vi "Drive_MP.vi"(8 "Backwards?":bool, 9 "Right Motor Name":string, 10 "Left Motor Name":string, 11 "Path Name":string) -> (0 "Time to Complete":dbl, 2 "Right Side Velocity Target":dbl, 3 "Left Side Velocity Target":dbl)   [LabVIEW 2020]
uses:
  <vilib>/Rock Robotics/WPI/ThirdParty/REV Robotics/REVLib/Typedef/Spark MAX Control Type.ctl
  <vilib>/Utility/file.llb/Read Delimited Spreadsheet (DBL).vi
panel:
  out "Measured Velocity":dbl
  out "Loop Iteration":dbl
  out "Velocity Target":dbl
  out "all rows":dbl[][](array[numeric])
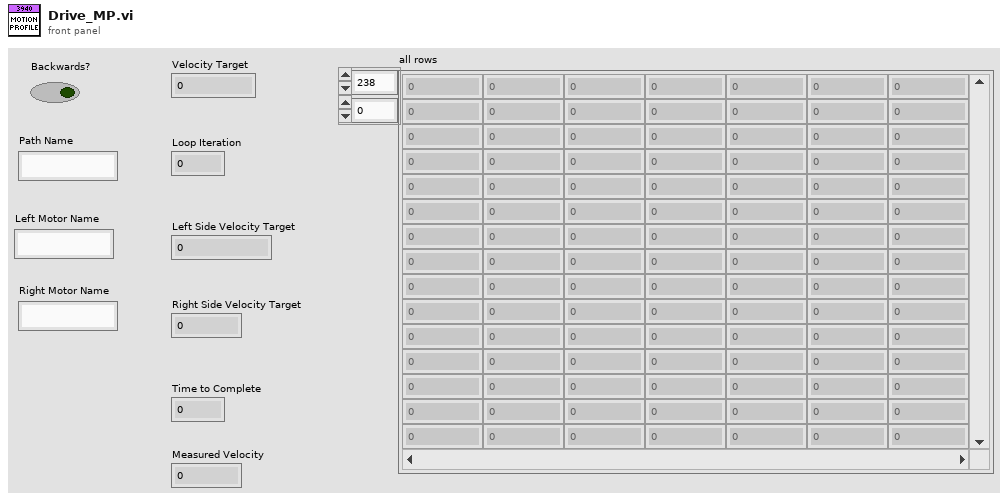
[diagram p1: front panel]
types:
  T1 = typedef "Spark MAX Control Type.ctl" = enum16{"Percent VBus", "Voltage", "Velocity", "Position", "Smart Motion", "Current", "Smart Velocity"}
  T2 = cluster{"P Gain":dbl, "I Gain":dbl, "D Gain":dbl, "F Gain":dbl, "I Zone":dbl, "Min Output":dbl, "Max Output":dbl}
  T3 = typedef "WPI_MotorControlDeviceRef.ctl" = cluster{"DeviceStatus":errorcluster, "Type":T4, "PWM":cluster{"PWM Channel":T5, "DeadBand":T6}, "CAN":cluster{"Device Number":u8, "SetOutput VI Ref":variant, "GetOutput VI Ref":variant, "Enable VI Ref":variant, "Disable VI Ref":variant, "Data":variant}, "Invert":bool, "DIO PWM":cluster{"PWM \"Enable\" Channel":T5, "DIOChannel":T7, "PWM Rate":dbl}}
  T4 = typedef "WPI_MotorControlType.ctl" = enum16{"PWM", "CAN", "DIO PWM"}
  T5 = typedef "FPGA_DIOPWMChannel.ctl" = enum8{"PWM 0", "PWM 1", "PWM 2", "PWM 3", "PWM 4", "PWM 5", "PWM 6", "PWM 7", "PWM 8", "PWM 9", "PWM MXP 0", "PWM MXP 1", "PWM MXP 2", "PWM MXP 3", "PWM MXP 4", "PWM MXP 5", "PWM MXP 6", "PWM MXP 7", "PWM MXP 8", "PWM MXP 9", "Invalid"}
  T6 = typedef "WPI_PWMDeadband.ctl" = cluster{"Name":string, "maxPositivePwm":i32, "minPositivePwm":i32, "centerPwm":i32, "maxNegativePwm":i32, "minNegativePwm":i32, "angularRange":u16}
  T7 = typedef "FPGA_DIOChannel.ctl" = enum8{"DIO 0", "DIO 1", "DIO 2", "DIO 3", "DIO 4", "DIO 5", "DIO 6", "DIO 7", "DIO 8", "DIO 9", "DIO MXP 0", "DIO MXP 1", "DIO MXP 2", "DIO MXP 3", "DIO MXP 4", "DIO MXP 5", "DIO MXP 6", "DIO MXP 7", "DIO MXP 8", "DIO MXP 9", "DIO MXP 10", "DIO MXP 11", "DIO MXP 12", "DIO MXP 13", "DIO MXP 14", "DIO MXP 15", "SPI Port CS1", "SPI Port CS2", "SPI Port CS3", "SPI Port MISO", "SPI Port MOSI", "Invalid"}
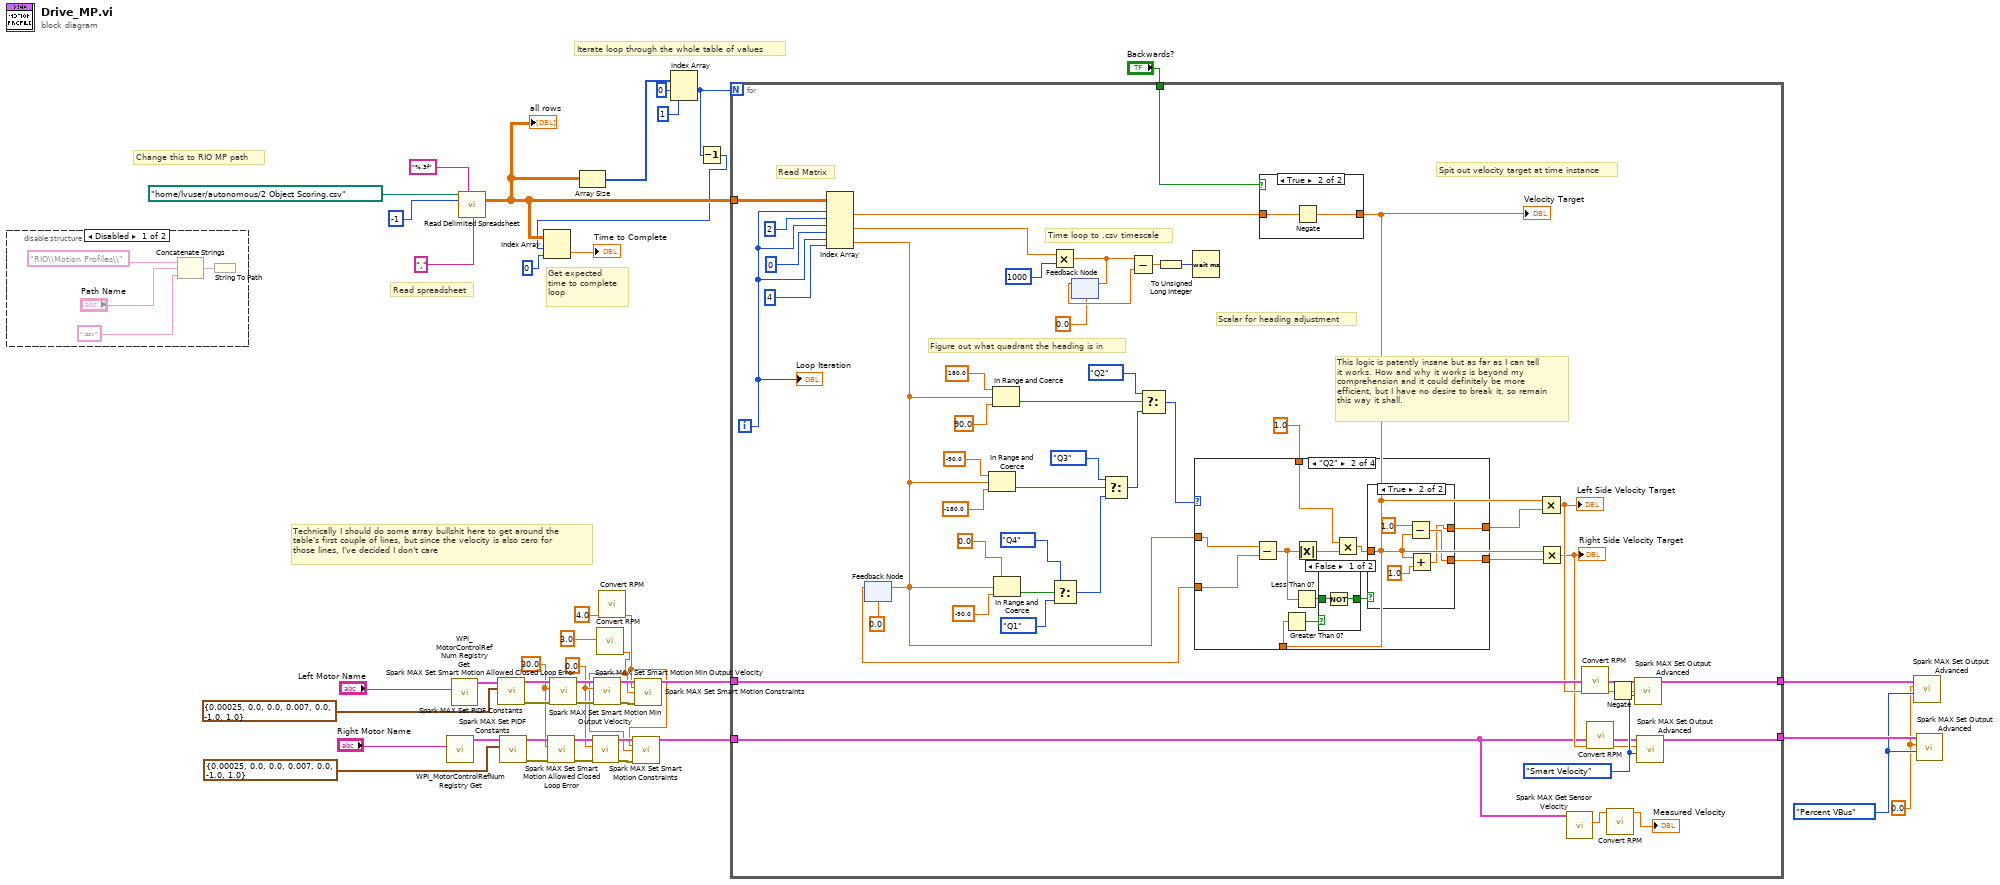
[diagram p0: block diagram]
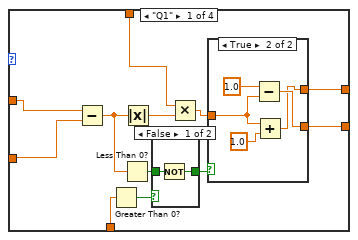
[diagram p4: hidden frame]
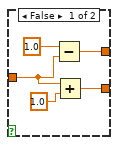
[diagram p6: hidden frame]
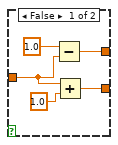
[diagram p8: hidden frame]
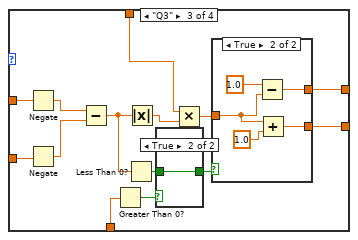
[diagram p9: hidden frame]
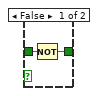
[diagram p10: hidden frame]
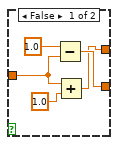
[diagram p11: hidden frame]
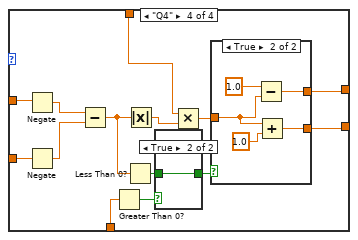
[diagram p12: hidden frame]
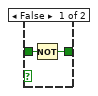
[diagram p13: hidden frame]
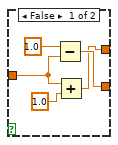
[diagram p14: hidden frame]
diagram:
  w3 = 0.0 ("Minimum Velocity Output")
  w4 = 30.0 ("Allowed Closed Loop Error")
  w21 = 0.0 ("Setpoint")
  w22 = Spark_MAX_Control_Type."Percent VBus" ("Control Mode")
  # "Get expected\ntime to complete\nloop"
  # "Change this to RIO MP path"
  # "Read spreadsheet"
  # "Iterate loop through the whole table of values"
  # "Technically I should do some array bullshit here to get around the\ntable's first couple of lines, but since the velocity is also zero for\nthose lines, I've decided I don't care"
  n1 = disable-structure shown="Disabled" {
    frame Disabled {
      n2 = Concatenate Strings("RIO\\Motion Profiles\\", "Path Name", ".csv") -> (w47:string)
      n3 = String To Path(string=w47) -> ()  [unwired: 1 out]
    }
    frame Enabled {
    }
  }
  n4 = call <vilib>:"WPI_MotorControlRefNum Registry Get.vi"("refnum name"="Right Motor Name") -> ("MotorControlDevRef"=w26:T3)  [unwired: 9 in, 1 out]
  n5 = call <vilib>:"WPI_MotorControlRefNum Registry Get.vi"("refnum name"="Left Motor Name") -> ("MotorControlDevRef"=w28:T3)  [unwired: 9 in, 1 out]
  n6 = call-poly <vilib>:"Read Delimited Spreadsheet.vi"("file path (dialog if empty)"=path "/home/lvuser/autonomous/2 Object Scoring.csv" ("file path (use dialog)"), "format (%.3f)"="%.3f", "number of rows (all:-1)"=-1, "delimiter (\\t)"="," ("delimiter (\\t)")) -> ("all rows"=w35:dbl[][])  [unwired: 6 in, 5 out]
  "all rows" <- w35
  n7 = call <vilib>:"Spark MAX Set PIDF Constants.vi"("PID Constants"=T2 {"P Gain"=0.00025, "I Gain"=0.0, "D Gain"=0.0, "F Gain"=0.007, "I Zone"=0.0, "Min Output"=-1.0, "Max Output"=1.0}, "MotorControlDeviceRef"=w28) -> ("error out"=w20:errorcluster, "MotorControlDeviceRef"=w19:T3)  [unwired: 8 in]
  n8 = call <vilib>:"Spark MAX Set PIDF Constants.vi"("PID Constants"=T2 {"P Gain"=0.00025, "I Gain"=0.0, "D Gain"=0.0, "F Gain"=0.007, "I Zone"=0.0, "Min Output"=-1.0, "Max Output"=1.0}, "MotorControlDeviceRef"=w26) -> ("error out"=w9:errorcluster, "MotorControlDeviceRef"=w10:T3)  [unwired: 8 in]
  n9 = call <vilib>:"Spark MAX Set Smart Motion Allowed Closed Loop Error.vi"("error in"=w9, "Allowed Closed Loop Error"=w4, "MotorControlDeviceRef"=w10) -> ("error out"=w12:errorcluster, "MotorControlDeviceRef"=w8:T3)  [unwired: 7 in]
  n10 = call <vilib>:"Spark MAX Set Smart Motion Allowed Closed Loop Error.vi"("error in"=w20, "Allowed Closed Loop Error"=w4, "MotorControlDeviceRef"=w19) -> ("error out"=w18:errorcluster, "MotorControlDeviceRef"=w17:T3)  [unwired: 7 in]
  n11 = Array Size(array=w35) -> (size(s)=w40:i32[])
  n12 = call <vilib>:"Spark MAX Set Smart Motion Min Output Velocity.vi"("error in"=w12, "Minimum Velocity Output"=w3, "MotorControlDeviceRef"=w8) -> ("error out"=w11:errorcluster, "MotorControlDeviceRef"=w7:T3)  [unwired: 7 in]
  n13 = call <vilib>:"Spark MAX Set Smart Motion Min Output Velocity.vi"("error in"=w18, "Minimum Velocity Output"=w3, "MotorControlDeviceRef"=w17) -> ("error out"=w15:errorcluster, "MotorControlDeviceRef"=w16:T3)  [unwired: 7 in]
  n14 = call "Convert RPM.vi"("Velocity (m/s)"=3.0) -> ("Velocity (RPM)"=w2:dbl)  [unwired: 9 in, 1 out]
  n15 = call "Convert RPM.vi"("Velocity (m/s)"=4.0) -> ("Velocity (RPM)"=w1:dbl)  [unwired: 9 in, 1 out]
  n16 = call <vilib>:"Spark MAX Set Smart Motion Constraints.vi"("MotorControlDeviceRef"=w7, "Max Velocity"=w1, "Max Acceleration"=w2, "error in"=w11) -> ("MotorControlDeviceRef"=w6:T3)  [unwired: 10 in, 1 out]
  n17 = call <vilib>:"Spark MAX Set Smart Motion Constraints.vi"("MotorControlDeviceRef"=w16, "Max Velocity"=w1, "Max Acceleration"=w2, "error in"=w15) -> ("MotorControlDeviceRef"=w5:T3)  [unwired: 10 in, 1 out]
  n18 = Index Array(array=w40, index #1=0 ("index"), index #2=1 ("index")) -> (element #1=w32:i32)  [unwired: 1 out]
  n19 = Decrement(x=w32) -> (x-1=w31:i32)
  n20 = Index Array(array=w35, index (row)=w31, index (col)=0 ("disabled index (col)")) -> (element=→"Time to Complete":dbl)
  n21 = for {
    N: w32 -> [_]
    tunnel: w35 -> [w96]
    tunnel: "Backwards?" -> [w60]
    tunnel: w5 -> [w59]
    tunnel: w6 -> [w51]
    tunnel: [w58] -> w24
    tunnel: [w57] -> w23
    i -> [w86]
    w56 = Spark_MAX_Control_Type."Smart Velocity" ("Control Mode")
    # "This logic is patently insane but as far as I can tell\nit works. How and why it works is beyond my\ncomprehension and it could definitely be more\nefficient, but I have no desire to break it, so remain\nthis way it shall."
    # "Scalar for heading adjustment"
    # "Figure out what quadrant the heading is in"
    # "Time loop to .csv timescale"
    # "Spit out velocity target at time instance"
    # "Read Matrix"
    n22 = Index Array(array=w96, index (row) #1=w86, index (col) #1=2 ("disabled index (col)"), index (row) #2=w86, index (col) #2=0 ("disabled index (col)"), index (row) #3=w86, index (col) #3=4 ("disabled index (col)")) -> (element #1=w62:dbl, element #2=w92:dbl, element #3=w67:dbl)
    n23 = feedback #1(0.0 ("Numeric")) -> (w68:dbl)
    n24 = feedback-in #1(w67) -> ()
    n25 = In Range and Coerce(upper limit=-90.0, x=w67, lower limit=-180.0) -> (In Range?=w78:bool)  [unwired: 1 out]
    n26 = In Range and Coerce(upper limit=180.0, x=w67, lower limit=90.0) -> (In Range?=w82:bool)  [unwired: 1 out]
    n27 = In Range and Coerce(upper limit=0.0, x=w67, lower limit=-90.0) -> (In Range?=w74:bool)  [unwired: 1 out]
    n28 = Multiply(x=w92, y=1000) -> (x*y=w88:dbl)
    n29 = Select(t=enum16{"Q1", "Q2", "Q3", "Q4"}."Q4", s=w74, f=enum16{"Q1", "Q2", "Q3", "Q4"}."Q1") -> (s? t:f=w71:enum16{"Q1", "Q2", "Q3", "Q4"})
    n30 = feedback #2(0.0) -> (w89:dbl)
    n31 = feedback-in #2(w88) -> ()
    n32 = Select(t=enum16{"Q1", "Q2", "Q3", "Q4"}."Q3", s=w78, f=w71) -> (s? t:f=w72:enum16{"Q1", "Q2", "Q3", "Q4"})
    n33 = Subtract(x=w88, y=w89) -> (x-y=w90:dbl)
    n34 = Select(t=enum16{"Q1", "Q2", "Q3", "Q4"}."Q2", s=w82, f=w72) -> (s? t:f=w69:enum16{"Q1", "Q2", "Q3", "Q4"})
    n35 = To Unsigned Long Integer(number=w90) -> (unsigned 32bit integer=w91:u32)
    n36 = Wait (ms)(milliseconds to wait=w91) -> ()  [unwired: 1 out]
    n37 = case shown="True" w60 {
      tunnel: w62 -> [w97 w99]
      tunnel: [w97 w98] -> w61
      frame False {
      }
      frame True {
        n38 = Negate(x=w99) -> (-x=w98:dbl)
      }
    }
    "Velocity Target" <- w61
    n39 = case shown="\"Q2\"" w69 {
      tunnel: w68 -> [w103 w125 w162 w178]
      tunnel: w67 -> [w104 w126 w163 w179]
      tunnel: [w100 w129 w158 w181] -> w65
      tunnel: [w101 w128 w157 w180] -> w64
      tunnel: 1.0 ("x") -> [w105 w130 w154 w182]
      tunnel: w61 -> [w102 w127 w153 w177]
      frame "Q1" {
        n40 = Subtract(x=w104, y=w103) -> (x-y=w111:dbl)
        n41 = Greater Than 0?(x=w102) -> (x > 0?=w108:bool)
        n42 = Less Than 0?(x=w111) -> (x < 0?=w107:bool)
        n43 = Absolute Value(x=w111) -> (abs(x)=w110:dbl)
        n44 = case shown="False" w108 {
          tunnel: w107 -> [w113 w114]
          tunnel: [w112 w114] -> w106
          frame False {
            n45 = Not(x=w113) -> (.not. x?=w112:bool)
          }
          frame True {
          }
        }
        n46 = Multiply(x=w105, y=w110) -> (x*y=w109:dbl)
        n47 = case shown="True" w106 {
          tunnel: w109 -> [w117 w121]
          tunnel: [w116 w120] -> w100
          tunnel: [w115 w122] -> w101
          frame False {
            n48 = Subtract(x=1.0, y=w117) -> (x-y=w116:dbl)
            n49 = Add(x=w117, y=1.0) -> (x+y=w115:dbl)
          }
          frame True {
            n50 = Subtract(x=1.0, y=w121) -> (x-y=w122:dbl)
            n51 = Add(x=w121, y=1.0) -> (x+y=w120:dbl)
          }
        }
      }
      frame "Q2" {
        n52 = Subtract(x=w126, y=w125) -> (x-y=w136:dbl)
        n53 = Greater Than 0?(x=w127) -> (x > 0?=w133:bool)
        n54 = Less Than 0?(x=w136) -> (x < 0?=w132:bool)
        n55 = Absolute Value(x=w136) -> (abs(x)=w135:dbl)
        n56 = case shown="False" w133 {
          tunnel: w132 -> [w138 w139]
          tunnel: [w137 w139] -> w131
          frame False {
            n57 = Not(x=w138) -> (.not. x?=w137:bool)
          }
          frame True {
          }
        }
        n58 = Multiply(x=w130, y=w135) -> (x*y=w134:dbl)
        n59 = case shown="True" w131 {
          tunnel: w134 -> [w142 w146]
          tunnel: [w141 w145] -> w129
          tunnel: [w140 w147] -> w128
          frame False {
            n60 = Subtract(x=1.0, y=w142) -> (x-y=w141:dbl)
            n61 = Add(x=w142, y=1.0) -> (x+y=w140:dbl)
          }
          frame True {
            n62 = Subtract(x=1.0, y=w146) -> (x-y=w147:dbl)
            n63 = Add(x=w146, y=1.0) -> (x+y=w145:dbl)
          }
        }
      }
      frame "Q3" {
        n64 = Negate(x=w163) -> (-x=w161:dbl)
        n65 = Negate(x=w162) -> (-x=w160:dbl)
        n66 = Subtract(x=w161, y=w160) -> (x-y=w159:dbl)
        n67 = Greater Than 0?(x=w153) -> (x > 0?=w152:bool)
        n68 = Less Than 0?(x=w159) -> (x < 0?=w151:bool)
        n69 = Absolute Value(x=w159) -> (abs(x)=w156:dbl)
        n70 = case shown="True" w152 {
          tunnel: w151 -> [w165 w166]
          tunnel: [w164 w166] -> w150
          frame False {
            n71 = Not(x=w165) -> (.not. x?=w164:bool)
          }
          frame True {
          }
        }
        n72 = Multiply(x=w154, y=w156) -> (x*y=w155:dbl)
        n73 = case shown="True" w150 {
          tunnel: w155 -> [w168 w174]
          tunnel: [w167 w173] -> w158
          tunnel: [w169 w172] -> w157
          frame False {
            n74 = Subtract(x=1.0, y=w168) -> (x-y=w169:dbl)
            n75 = Add(x=w168, y=1.0) -> (x+y=w167:dbl)
          }
          frame True {
            n76 = Subtract(x=1.0, y=w174) -> (x-y=w173:dbl)
            n77 = Add(x=w174, y=1.0) -> (x+y=w172:dbl)
          }
        }
      }
      frame "Q4" {
        n78 = Negate(x=w179) -> (-x=w190:dbl)
        n79 = Negate(x=w178) -> (-x=w189:dbl)
        n80 = Subtract(x=w190, y=w189) -> (x-y=w188:dbl)
        n81 = Greater Than 0?(x=w177) -> (x > 0?=w185:bool)
        n82 = Less Than 0?(x=w188) -> (x < 0?=w184:bool)
        n83 = Absolute Value(x=w188) -> (abs(x)=w187:dbl)
        n84 = case shown="True" w185 {
          tunnel: w184 -> [w192 w193]
          tunnel: [w191 w193] -> w183
          frame False {
            n85 = Not(x=w192) -> (.not. x?=w191:bool)
          }
          frame True {
          }
        }
        n86 = Multiply(x=w182, y=w187) -> (x*y=w186:dbl)
        n87 = case shown="True" w183 {
          tunnel: w186 -> [w195 w201]
          tunnel: [w194 w200] -> w181
          tunnel: [w196 w199] -> w180
          frame False {
            n88 = Subtract(x=1.0, y=w195) -> (x-y=w196:dbl)
            n89 = Add(x=w195, y=1.0) -> (x+y=w194:dbl)
          }
          frame True {
            n90 = Subtract(x=1.0, y=w201) -> (x-y=w200:dbl)
            n91 = Add(x=w201, y=1.0) -> (x+y=w199:dbl)
          }
        }
      }
    }
    n92 = Multiply(x=w61, y=w65) -> (x*y=w55:dbl)
    "Left Side Velocity Target" <- w55
    n93 = Multiply(x=w61, y=w64) -> (x*y=w52:dbl)
    "Right Side Velocity Target" <- w52
    n94 = call <vilib>:"Spark MAX Get Sensor Velocity.vi"("MotorControlDevRef in"=w51) -> ("Sensor Velocity"=w49:dbl)  [unwired: 7 in, 3 out]
    n95 = call "Convert RPM.vi"("Velocity (m/s)"=w55) -> ("Velocity (RPM)"=w54:dbl)  [unwired: 9 in, 1 out]
    n96 = call "Convert RPM.vi"("Velocity (m/s)"=w52) -> ("Velocity (RPM)"=w53:dbl)  [unwired: 9 in, 1 out]
    n97 = call "Convert RPM.vi"("Velocity (RPM)"=w49) -> ("Velocity (m/s)"=→"Measured Velocity":dbl)  [unwired: 9 in, 1 out]
    n98 = Negate(x=w54) -> (-x=w50:dbl)
    n99 = call <vilib>:"Spark MAX Set Output Advanced.vi"("Control Mode"=w56, "Setpoint"=w50, "MotorControlDevRef"=w59) -> ("MotorControlDevRef"=w58:T3)  [unwired: 7 in, 1 out]
    n100 = call <vilib>:"Spark MAX Set Output Advanced.vi"("Control Mode"=w56, "Setpoint"=w53, "MotorControlDevRef"=w51) -> ("MotorControlDevRef"=w57:T3)  [unwired: 7 in, 1 out]
    "Loop Iteration" <- w86
  }
  n101 = call <vilib>:"Spark MAX Set Output Advanced.vi"("Control Mode"=w22, "Setpoint"=w21, "MotorControlDevRef"=w24) -> ()  [unwired: 7 in, 2 out]
  n102 = call <vilib>:"Spark MAX Set Output Advanced.vi"("Control Mode"=w22, "Setpoint"=w21, "MotorControlDevRef"=w23) -> ()  [unwired: 7 in, 2 out]
